vi "Read call chain.vi"(8 "error in (no error)":errorcluster, 11 "LogRecord in":refnum<class "LogRecord.lvclass">) -> (0 "error out":errorcluster, 2 "call chain":string[](array[string]), 3 "LogRecord out":refnum<class "LogRecord.lvclass">)   [LabVIEW 2024, in "LogRecord.lvclass"]
uses:
  LogRecord.lvclass
  LogRecord.lvclass/LogRecord.ctl
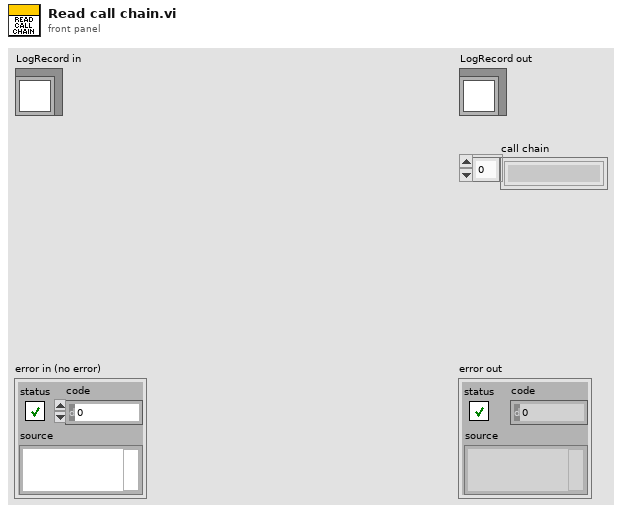
[diagram p1: front panel]
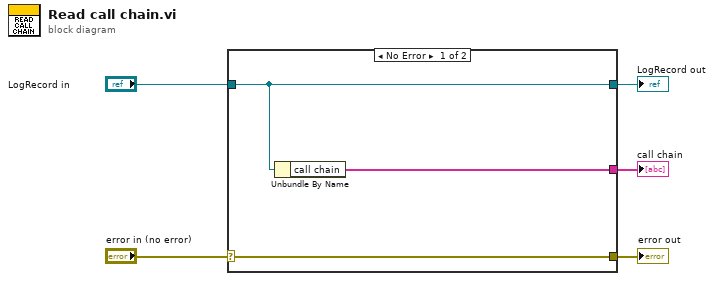
[diagram p0: block diagram]
diagram:
  n1 = case shown="No Error" "error in (no error)" {
    selector: "error in (no error)" -> [w8 w9]
    tunnel: [w8 w9] -> w4
    tunnel: [w7 w10] -> w2
    tunnel: "LogRecord in" -> [w7 w10]
    tunnel: [w6 _] -> w1
    frame No Error {
      n2 = Unbundle By Name(w7) -> ("call chain"=w6:string[])
    }
    frame Error {
    }
  }
  "error out" <- w4
  "LogRecord out" <- w2
  "call chain" <- w1
